vi "PAN_ChkResp.vi"(7 "cmdID  in":string, 10 "resp in":string, 11 "source":string) -> (2 "resp out":string)   [LabVIEW 2016]
uses:
  Modules/DBSHAND/private/vis/DatabaseHand_Element_Set(string).vi
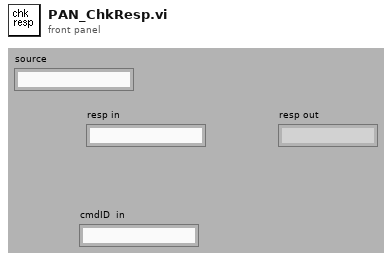
[diagram p1: front panel]
types:
  T1 = typedef "DatabaseHand_RefNum.ctl" = refnum<vi>
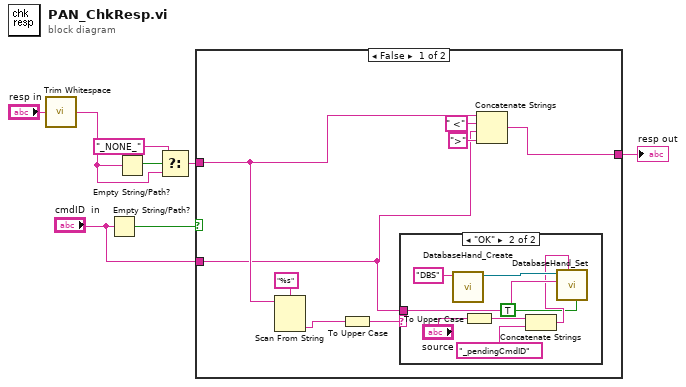
[diagram p0: block diagram]
diagram:
  n1 = call <vilib>:"Trim Whitespace.vi"("string"="resp in") -> ("trimmed string"=w5:string)  [unwired: 1 in]
  n2 = Empty String/Path?(string/path="cmdID  in") -> (empty?=w4:bool)
  n3 = Empty String/Path?(string/path=w5) -> (empty?=w8:bool)
  n4 = Select(t="_NONE_", s=w8, f=w5) -> (s? t:f=w3:string)
  n5 = case shown="False" w4 {
    tunnel: w3 -> [w13 w25]
    tunnel: [w14 w25] -> w2
    tunnel: "cmdID  in" -> [w9 _]
    frame False {
      n6 = Scan From String(format string="%s", input string=w13) -> (output 1=w11:string)  [unwired: 2 in, 4 out]
      n7 = To Upper Case(1:w11) -> (0:w10:string)
      n8 = case shown="\"OK\"" w10 {
        tunnel: w9 -> [_ w22]
        frame "False", Default {
        }
        frame "OK" {
          n9 = call "DatabaseHand_Create.vi"("Name"="DBS") -> ("Database RefNum out"=w24:T1)  [unwired: 1 in, 9 out]
          n10 = To Upper Case(1:"source") -> (0:w18:string)
          n11 = Concatenate Strings(w18, "_pendingCmdID" ("name")) -> (w19:string)
          n12 = call-poly "DatabaseHand_Set.vi"("enqueue? (F)"=TRUE, "name"=w19, "value"=w22, "Database RefNum in"=w24) -> ()  [unwired: 4 in, 4 out]
        }
      }
      n13 = Concatenate Strings(w13, " <" ("string"), w9, ">" ("string")) -> (w14:string)
    }
    frame True {
    }
  }
  "resp out" <- w2
